vi "SPI_Get_GPIOs.vi"(5 "Handle":u32) -> (0 "High IO Values":cluster{bool, bool, bool, bool}, 2 "FTC_Status":u32)   [LabVIEW 2010]
uses:
  WINNT/system32/FTCSPI.dll
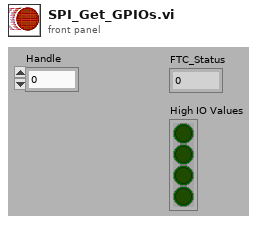
[diagram p1: front panel]
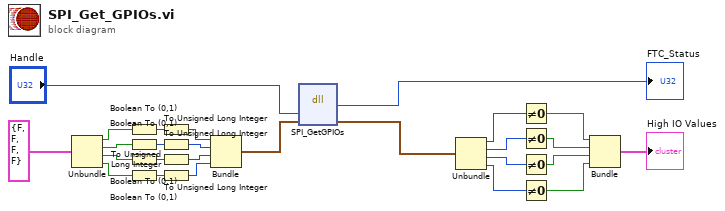
[diagram p0: block diagram]
diagram:
  n1 = Unbundle(cluster{bool, bool, bool, bool} {FALSE, FALSE, FALSE, FALSE} ("output cluster")) -> (w20:bool, w19:bool, w18:bool, w17:bool)
  n2 = Boolean To (0,1)(Boolean=w20) -> (0, 1=w24:i16)
  n3 = Boolean To (0,1)(Boolean=w19) -> (0, 1=w21:i16)
  n4 = Boolean To (0,1)(Boolean=w18) -> (0, 1=w22:i16)
  n5 = Boolean To (0,1)(Boolean=w17) -> (0, 1=w23:i16)
  n6 = To Unsigned Long Integer(number=w24) -> (unsigned 32bit integer=w15:u32)
  n7 = To Unsigned Long Integer(number=w21) -> (unsigned 32bit integer=w14:u32)
  n8 = To Unsigned Long Integer(number=w22) -> (unsigned 32bit integer=w12:u32)
  n9 = To Unsigned Long Integer(number=w23) -> (unsigned 32bit integer=w13:u32)
  n10 = Bundle(w15, w14, w12, w13) -> (w2:cluster{u32, u32, u32, u32})  [unwired: 1 in]
  n11 = dll-call lib="C:/Users/WINNT/system32/FTCSPI.dll" fn="SPI_GetGPIOs"("Handle"="Handle", w2) -> ("FTC_Status"=→"FTC_Status":u32, w1:cluster{u32, u32, u32, u32})  [unwired: 4 in, 2 out]
  n12 = Unbundle(w1) -> (w6:u32, w5:u32, w4:u32, w3:u32)
  n13 = Not Equal To 0?(x=w6) -> (x != 0?=w11:bool)
  n14 = Not Equal To 0?(x=w5) -> (x != 0?=w10:bool)
  n15 = Not Equal To 0?(x=w4) -> (x != 0?=w9:bool)
  n16 = Not Equal To 0?(x=w3) -> (x != 0?=w8:bool)
  n17 = Bundle(w11, w10, w9, w8) -> (→"High IO Values":cluster{bool, bool, bool, bool})  [unwired: 1 in]
